vi "Get Enum Details from Type String.vi"(11 "type string IN":i16[](array[numeric])) -> (1 "Item Count":i16, 2 "Item Strings":string[](array[string]), 3 "Name":string)   [LabVIEW 2014, in "hse-misc.lvlib"]
uses:
  hse-misc.lvlib
panel:
  out "Type String (U8)":u8[](array[numeric])
  out "type string (I16)":i16[](array[numeric])
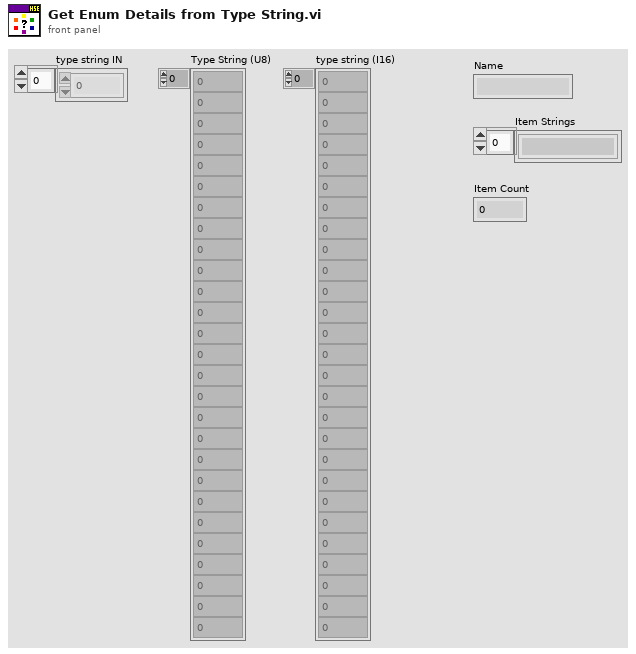
[diagram p1: front panel]
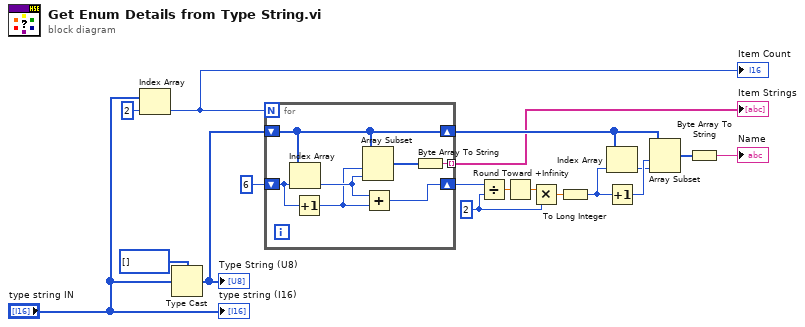
[diagram p0: block diagram]
diagram:
  w17 = 2 ("y")
  n1 = Index Array(array="type string IN", index=2) -> (element=w15:i16)
  "Item Count" <- w15
  n2 = Type Cast(type=u8[] [], x="type string IN") -> (*(type *) &x=w5:u8[])
  "Type String (U8)" <- w5
  n3 = for {
    N: w15 -> [_]
    shift-right: [w24] -> w7
    shift-left: 6 -> [w21]
    tunnel: [w22] -> w6 mode=indexing
    shift-right: [w19] -> w9
    shift-left: w5 -> [w19]
    n4 = Index Array(array=w19, index=w21) -> (element=w25:u8)
    n5 = Increment(x=w21) -> (x+1=w20:i32)
    n6 = Array Subset(array=w19, index=w20, length=w25) -> (w23:u8[])
    n7 = Add(x=w25, y=w20) -> (x+y=w24:i32)
    n8 = Byte Array To String(unsigned byte array=w23) -> (string=w22:string)
  }
  "Item Strings" <- w6
  n9 = Divide(x=w7, y=w17) -> (x/y=w8:dbl)
  n10 = Round Toward +Infinity(x=w8) -> (ceil(x): smallest int >= x=w11:dbl)
  n11 = Multiply(x=w11, y=w17) -> (x*y=w16:dbl)
  n12 = To Long Integer(number=w16) -> (32bit integer=w18:i32)
  n13 = Index Array(array=w9, index=w18) -> (element=w10:u8)
  n14 = Increment(x=w18) -> (x+1=w12:i32)
  n15 = Array Subset(array=w9, index=w12, length=w10) -> (w13:u8[])
  n16 = Byte Array To String(unsigned byte array=w13) -> (string=→"Name":string)
  "type string (I16)" <- "type string IN"
